vi "_PC_Pub_Boolean2DBL.vi"(1 "Boolean array":bool[](array[boolean])) -> (0 "DBL":dbl)   [LabVIEW 2018]
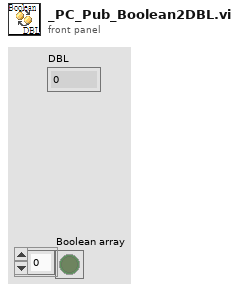
[diagram p1: front panel]
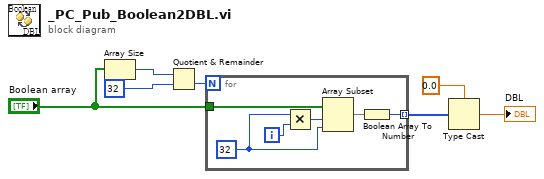
[diagram p0: block diagram]
diagram:
  n1 = Array Size(array="Boolean array") -> (size(s)=w4:i32)
  n2 = Quotient & Remainder(x=w4, y=32) -> (floor(x/y)=w2:i32)  [unwired: 1 out]
  n3 = for {
    N: w2 -> [_]
    tunnel: "Boolean array" -> [w13]
    tunnel: [w8] -> w7 mode=indexing
    i -> [w12]
    w10 = 32 ("x")
    n4 = Multiply(x=w10, y=w12) -> (x*y=w11:i32)
    n5 = Array Subset(array=w13, index=w11, length=w10) -> (w9:bool[])
    n6 = Boolean Array To Number(Boolean array=w9) -> (number=w8:u32)
  }
  n7 = Type Cast(type=0.0, x=w7) -> (*(type *) &x=→"DBL":dbl)
